vi "COMI FC Select Gate.vi"(9 "nGateIndex":i32, 10 "ch":i32, 11 "hDevice":u32) -> (3 "hDevice out":u32)   [LabVIEW 2017, in "Comidll.lvlib"]
doc: "void (COMI_FC_SelectGate) (HANDLE hDevice, int ch, int nGateIndex);"
uses:
  <userlib>/Comidll/Comidll.lvlib
  <userlib>/Comidll/Comidll.dll
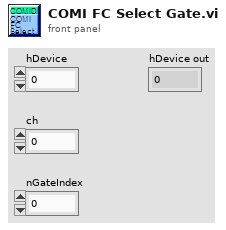
[diagram p1: front panel]
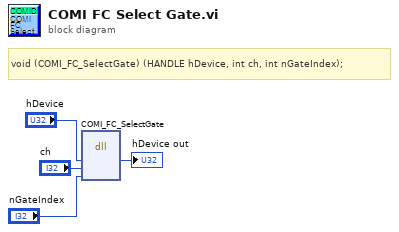
[diagram p0: block diagram]
diagram:
  # "void\t(COMI_FC_SelectGate) (HANDLE hDevice, int ch, int nGateIndex);"
  n1 = dll-call lib="C:/Program Files/National Instruments/LabVIEW 2017/user.lib/Comidll/Comidll.*" fn="COMI_FC_SelectGate"("hDevice"="hDevice", "ch"="ch", "nGateIndex"="nGateIndex") -> ("hDevice"=→"hDevice out":u32)  [unwired: 6 in, 2 out]
